vi "Validate Flash.vi"(8 "error in":errorcluster, 11 "MPLab in":refnum<class "MPLab.lvclass">) -> (0 "error out":errorcluster, 1 "Failure Message":string, 2 "Success?":bool, 3 "MPLab out":refnum<class "MPLab.lvclass">)   [LabVIEW 2018, in "MPLab.lvlib" / "MPLab.lvclass"]
uses:
  MPLab.lvclass
  MPLab.lvclass/MPLab.ctl
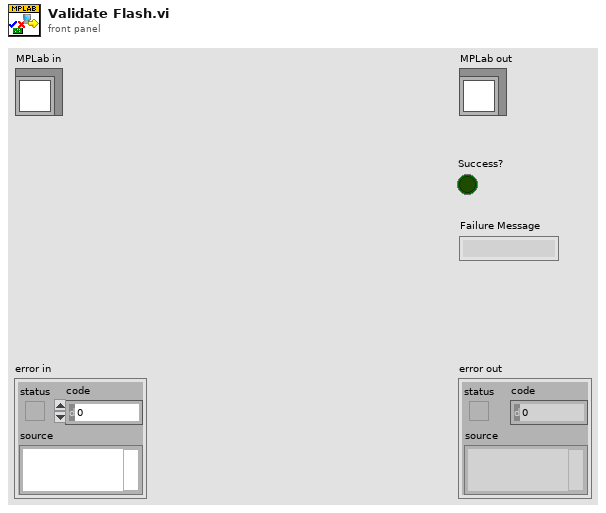
[diagram p1: front panel]
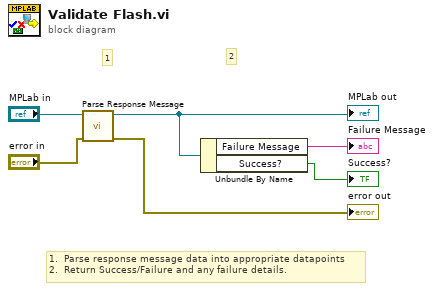
[diagram p0: block diagram]
diagram:
  # "1.  Parse response message data into appropriate datapoints\n2.  Return Success/Failure and any failure details."
  # "2"
  # "1"
  n1 = call "Parse Response Message.vi"("error in"="error in", "MPLab in"="MPLab in") -> ("error out"=→"error out":errorcluster, "MPLab out"=w3:refnum<class "MPLab.lvclass">)  [unwired: 8 in]
  "MPLab out" <- w3
  n2 = Unbundle By Name(w3) -> ("Failure Message"=→"Failure Message":string, "Success?"=→"Success?":bool)
